vi "DFD FXP NStage MRate Simulation (I32).vi"(5 "input range":dbl=1.0, 7 "init? (T)":bool=TRUE, 8 "error in (no error)":errorcluster, 10 "multirate filters":T1[](array[typedef]) {"mMRate_SumWl" min=1 max=32 step=1; "mMRate_InputIwl" min=1 max=32 step=1; "mMRate_GainWl" min=1 max=32 step=1; "mMRate_OutputWl" min=1 max=32 step=1; "mMRate_InputWl" min=1 max=32 step=1; "mMRate_CoefWl" min=1 max=32 step=1; "mMRate_Mode" items=["Default"=-1, "No Rate Change"=0, "Interpolation"=1, "Decimation"=2, "Interpolated"=3, "Rational"=4]}, 11 "signal in":i32[](array[numeric])) -> (0 "error out":errorcluster, 2 "integer signal out":i32[](array[numeric]), 3 "DBL signal out":dbl[](array[numeric]))   [LabVIEW 2017, in "NI_DigFilterLicensed.lvlib"]
doc: "Simulates the filtering process of a fixed-point multistage multirate filter continuously. Wire data to the <B>signal in</B> input to determine the polymorphic instance to use or manually select the instance."
uses:
  <vilib>/addons/Digital Filter Design/NI_DigFilterLicensed.lvlib
  <vilib>/addons/Digital Filter Design/_Objects.llb/DFD Multirate Filter Obj.ctl
  <vilib>/addons/Digital Filter Design/_Objects.llb/DFD Multirate Mode.ctl
  <vilib>/addons/Digital Filter Design/_Objects.llb/DFD Coef Norm Type.ctl
  <vilib>/addons/Digital Filter Design/_Objects.llb/DFD Round-off Mode.ctl
  <vilib>/addons/Digital Filter Design/_Objects.llb/DFD FXP MRate Multiply Mode.ctl
  <vilib>/addons/Digital Filter Design/_Misc.llb/dfd_Error Handlers (Single).vi
  <vilib>/addons/Digital Filter Design/NI_DigFilter_FXP.lvlib
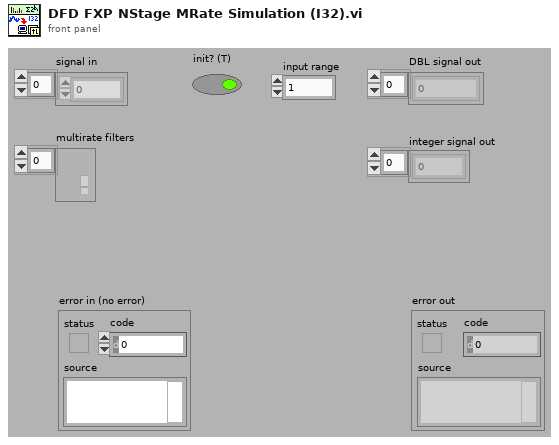
[diagram p1: front panel]
types:
  T1 = typedef "NI_DigFilterLicensed.lvlib/DFD Multirate Filter Obj.ctl" = cluster{"mMRate_Structure":enum16{"CIC", "FIR", "IIR", "Lattice"}, "mMRate_Mode":T2, "mMRate_Factor":i32, "mMRate_FIRParams":cluster{"mMRate_FIR_H":dbl[], "mMRate_FIR_IsNyquist?":bool, "mMRate_FIR_IsSymmetric?":bool}, "mMRate_CICParams":cluster{"mMRate_CIC_#Stage":i32, "mMRate_CIC_Lag":i32, "mMRate_CIC_Type":enum16{"Lowpass", "Highpass"}}, "mMRate_Order":i32, "mMRate_Version":string, "mMRate_Comments":string, "mMRate_RationalFactor":cluster{"mMRate_L":i32, "mMRate_M":i32}, "mMRate_Fs":dbl, "mMRate_Quantized?":bool, "mMRate_QFilterGain":dbl, "mMRate_CoefWl":i16, "mMRate_Scaling":cluster{"mMRate_ScaleByPowerOf2?":bool, "mMRate_ScaleType":T3}, "mMRate_InputWl":i16, "mMRate_OutputWl":i16, "mMRate_OutputMode":T4, "mMRate_MultMode":T5, "mMRate_BitPruning":bool, "mMRate_GainWl":i16, "mMRate_OutputFwl":i16, "mMRate_SumIwl":i16, "mMRate_InputIwl ":i16, "mMRate_SumWl":i16, "mMRate_CoefIwl":i16}
  T2 = typedef "NI_DigFilterLicensed.lvlib/DFD Multirate Mode.ctl" = i16
  T3 = typedef "NI_DigFilterLicensed.lvlib/DFD Coef Norm Type.ctl" = enum16{"No Norm", "Time Domain 1-Norm", "Time Domain 2-Norm", "Time Domain Inf-Norm"}
  T4 = typedef "NI_DigFilterLicensed.lvlib/DFD Round-off Mode.ctl" = enum16{"Nearest", "Truncation"}
  T5 = typedef "NI_DigFilterLicensed.lvlib/DFD FXP MRate Multiply Mode.ctl" = enum16{"Truncated", "Full"}
  T6 = typedef "dfd_FXP MRate Simu State.ctl" = cluster{"acc1":T7[], "acc2":T7[], "FIR state":i64[], "next phase":i32}
  T7 = typedef "dfd_Integer I160.ctl" = cluster{"Hi [I32]":i32, "Lo3 [U32]":u32, "Lo2 [U32]":u32, "Lo1 [U32]":u32, "Lo0 [U32]":u32}
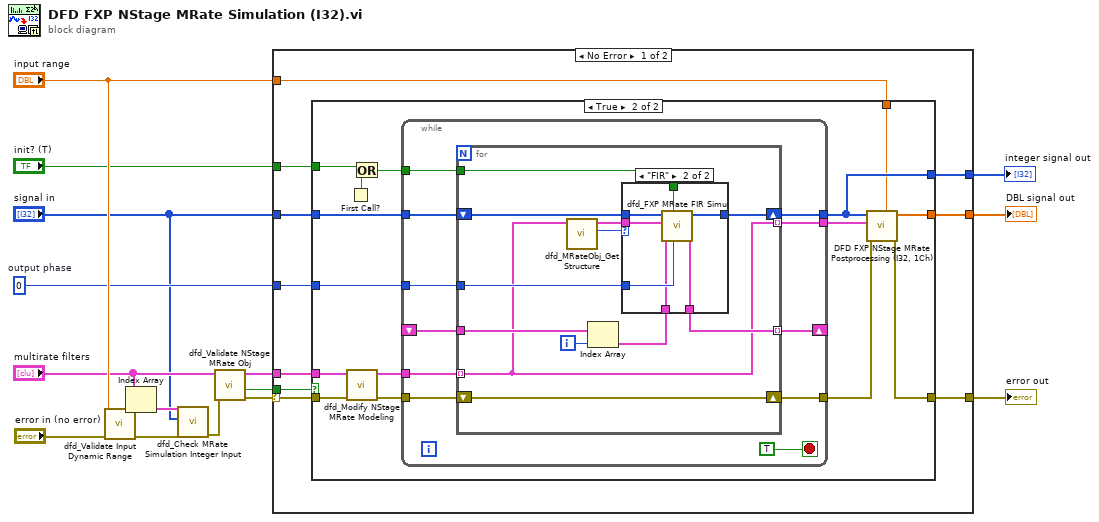
[diagram p0: block diagram]
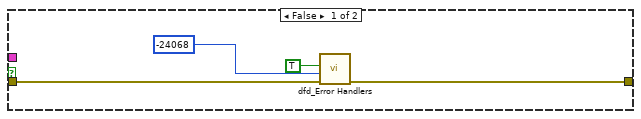
[diagram p2: hidden frame]
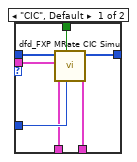
[diagram p3: hidden frame]
diagram:
  w8 = 0  # output phase
  n1 = call <vilib>:"dfd_Validate Input Dynamic Range.vi"("error in (no error)"="error in (no error)", "input range"="input range") -> ("error out"=w7:errorcluster)  [unwired: 9 out]
  n2 = Index Array(array="multirate filters") -> (element=w5:T1)  [unwired: 1 in]
  n3 = call <vilib>:"dfd_Check MRate Simulation Integer Input.vi"("error in (no error)"=w7, "signal in"="signal in", "multirate filter"=w5) -> ("error out"=w6:errorcluster)  [unwired: 8 out]
  n4 = call <vilib>:"dfd_Validate NStage MRate Obj.vi"("error in"=w6, "multirate filters"="multirate filters") -> ("error out"=w1:errorcluster, "is valid FXP?"=w12:bool, "dup multirate filters"=w11:T1[])  [unwired: 7 out]
  n5 = case shown="No Error" w1 {
    selector: w1 -> [w16 w82]
    tunnel: [w25 _] -> w15
    tunnel: [w24 w82] -> w14
    tunnel: "input range" -> [w23 _]
    tunnel: w12 -> [w22 _]
    tunnel: w11 -> [w21 _]
    tunnel: [w20 _] -> w10
    tunnel: w8 -> [w19 _]
    tunnel: "init? (T)" -> [w18 _]
    tunnel: "signal in" -> [w17 _]
    frame No Error {
      n6 = case shown="True" w22 {
        tunnel: w17 -> [_ w44]
        tunnel: w23 -> [_ w33]
        tunnel: [_ w43] -> w25
        tunnel: [w26 w42] -> w24
        tunnel: w21 -> [_ w38]
        tunnel: w16 -> [w29 w36]
        tunnel: [_ w39] -> w20
        tunnel: w19 -> [_ w34]
        tunnel: w18 -> [_ w32]
        frame False {
          n7 = call-poly <vilib>:"dfd_Error Handlers.vi"("error in (no error)"=w29, "error code"=-24068 ("ERR_INVALID_FXP_MRATE"), "condition failed?"=TRUE) -> ("error out"=w26:errorcluster)  [unwired: 8 out]
        }
        frame True {
          n8 = First Call?() -> (First Call?: T/F=w31:bool)
          n9 = call <vilib>:"dfd_Modify NStage MRate Modeling.vi"("error in (no error)"=w36, "multirate filters in"=w38) -> ("error out"=w35:errorcluster, "multirate filters out"=w37:T1[])  [unwired: 8 out]
          n10 = Or(x=w32, y=w31) -> (x .or. y?=w30:bool)
          n11 = while {
            tunnel: w44 -> [w55]
            tunnel: [w54] -> w41
            tunnel: [w53] -> w40
            tunnel: [w52] -> w39
            tunnel: w37 -> [w51]
            tunnel: w35 -> [w50]
            tunnel: w34 -> [w49]
            tunnel: w30 -> [w47]
            shift-right: [w46] -> _
            shift-left: _ -> [w45]
            stop <- TRUE stop-if-true
            n12 = for {
              tunnel: [w56] -> w54 mode=indexing
              tunnel: w51 -> [w56] mode=indexing
              shift-right: [w66] -> w52
              shift-left: w55 -> [w67]
              shift-right: [w63] -> w53
              shift-left: w50 -> [w63]
              tunnel: w49 -> [w62]
              tunnel: w47 -> [w61]
              tunnel: [w60] -> w46 mode=indexing
              tunnel: w45 -> [w59]
              i -> [w58]
              n13 = call <vilib>:"dfd_MRateObj_Get Structure.vi"("multirate filter in"=w56) -> ("structure"=w65:enum16{"CIC", "FIR", "IIR", "Lattice"}, "dup multirate filter"=w64:T1)  [unwired: 9 out]
              n14 = Index Array(array=w59, index=w58) -> (element=w57:T6)
              n15 = case shown="\"FIR\"" w65 {
                tunnel: w64 -> [w71 w78]
                tunnel: w67 -> [w74 w81]
                tunnel: [w73 w80] -> w66
                tunnel: w62 -> [w72 w79]
                tunnel: w61 -> [w70 w77]
                tunnel: [w69 w75] -> w60
                tunnel: w57 -> [w68 w76]
                frame "CIC", Default {
                  n16 = call <vilib>:"dfd_FXP MRate CIC Simu.vi"("output phase"=w72, "init? (T)"=w70, "FXPMRateSimState in"=w68, "FXP CIC"=w71, "signal in"=w74) -> ("FXPMRateSimState out"=w69:T6, "signal out"=w73:i32[])  [unwired: 5 out]
                }
                frame "FIR" {
                  n17 = call <vilib>:"dfd_FXP MRate FIR Simu.vi"("output phase"=w79, "init? (T)"=w77, "FXPMRateSimState in"=w76, "multirate filter"=w78, "signal in"=w81) -> ("FXPMRateSimState out"=w75:T6, "signal out"=w80:i32[])  [unwired: 1 in, 4 out]
                }
              }
            }
          }
          n18 = call <vilib>:"DFD FXP NStage MRate Postprocessing (I32, 1Ch).vi"("input range"=w33, "error in (no error)"=w40, "multirate filters"=w41, "signal in"=w39) -> ("error out"=w42:errorcluster, "signal out"=w43:dbl[])  [unwired: 1 in, 5 out]
        }
      }
    }
    frame Error {
    }
  }
  "error out" <- w14
  "DBL signal out" <- w15
  "integer signal out" <- w10
